vi "DataPacker_Restart.vi"(9 "Max Queue Size (-1, unlimited)":i32, 10 "Override Max Event size (Data rate kb/s). Use MIDAS Default = 0":u32, 11 "stop":bool) -> ()   [LabVIEW 2018, in "feGEM DataPacker.lvlib"]
uses:
  feGEM DataPacker.lvlib
  DataPacker_Settings.ctl
  DataPacker_Commands.ctl
panel:
  out "# elements in queue":i32
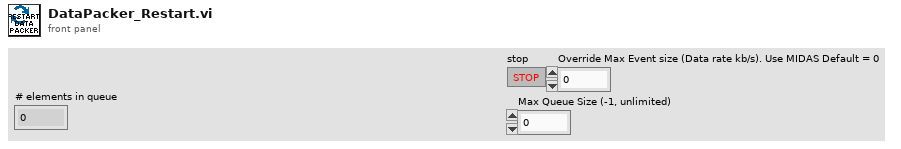
[diagram p1: front panel]
types:
  T1 = typedef "feGEM DataPacker.lvlib/DataPacker_Settings.ctl" = cluster{"Override Max Event size (Data rate kb/s). Use MIDAS Default = 0":u32, "MIDAS Server":string, "MIDAS Server Port":u16, "Max Queue Size (-1, unlimited)":i32, "DataPacker_Command":T2, "Caller VI":string[]}
  T2 = typedef "feGEM DataPacker.lvlib/DataPacker_Commands.ctl" = enum16{"Do Nothing", "Restart", "Stop"}
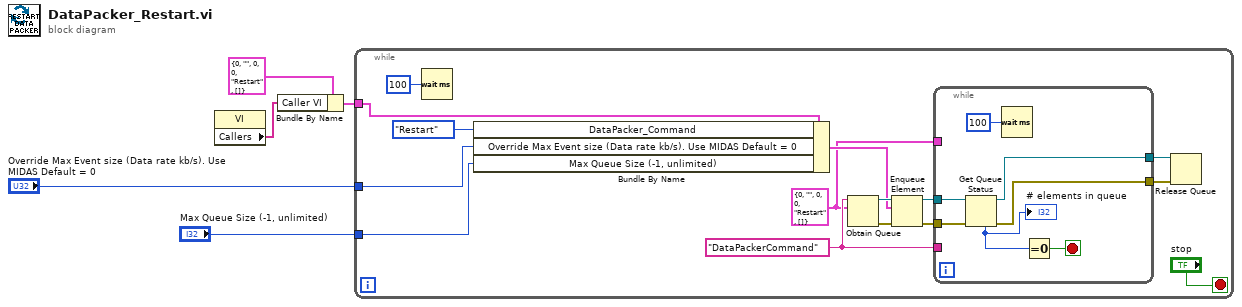
[diagram p0: block diagram]
diagram:
  n1 = property class="VI"() -> ("Callers"=w5:string[])  [unwired: 2 in, 2 out]
  n2 = Bundle By Name(cluster=T1 {"Override Max Event size (Data rate kb/s). Use MIDAS Default = 0"=0, "MIDAS Server"="", "MIDAS Server Port"=0, "Max Queue Size (-1, unlimited)"=0, "DataPacker_Command"=enum."Restart", "Caller VI"=[]} ("output cluster"), "Caller VI"=w5) -> (w3:T1)
  n3 = while {
    tunnel: w3 -> [w10]
    tunnel: "Override Max Event size (Data rate kb/s). Use MIDAS Default = 0" -> [w7]
    tunnel: "Max Queue Size (-1, unlimited)" -> [w6]
    stop <- "stop" stop-if-true
    w11 = T1 {"Override Max Event size (Data rate kb/s). Use MIDAS Default = 0"=0, "MIDAS Server"="", "MIDAS Server Port"=0, "Max Queue Size (-1, unlimited)"=0, "DataPacker_Command"=enum."Restart", "Caller VI"=[]} ("output cluster")
    w12 = "DataPackerCommand" ("name (unnamed)")
    n4 = Wait (ms)(milliseconds to wait=u32 100) -> ()  [unwired: 1 out]
    n5 = Bundle By Name(cluster=w10, "DataPacker_Command"=DataPacker_Commands."Restart", "Override Max Event size (Data rate kb/s). Use MIDAS Default = 0"=w7, "Max Queue Size (-1, unlimited)"=w6) -> (w17:T1)
    n6 = Obtain Queue(name (unnamed)=w12, element data type=w11) -> (queue out=w18:refnum<queue>, error out=w19:errorcluster)  [unwired: 3 in, 1 out]
    n7 = Enqueue Element(queue=w18, element=w17, error in (no error)=w19) -> (queue out=w16:refnum<queue>, error out=w15:errorcluster)  [unwired: 1 in, 1 out]
    n8 = while {
      tunnel: w12 -> [_]
      tunnel: w11 -> [_]
      tunnel: w16 -> [w27]
      tunnel: w15 -> [w26]
      tunnel: [w25] -> w13
      tunnel: [w24] -> w14
      stop <- w22 stop-if-true
      n9 = Get Queue Status(queue=w27, error in (no error)=w26) -> (queue out=w25:refnum<queue>, error out=w24:errorcluster, # elements in queue=w23:i32)  [unwired: 1 in, 5 out]
      "# elements in queue" <- w23
      n10 = Wait (ms)(milliseconds to wait=u32 100) -> ()  [unwired: 1 out]
      n11 = Equal To 0?(x=w23) -> (x = 0?=w22:bool)
    }
    n12 = Release Queue(queue=w13, error in (no error)=w14) -> ()  [unwired: 1 in, 3 out]
  }
